vi "ClimbSequencer.vi"(7 "Reinit":bool) -> (0 "Climber Climbing":bool, 1 "Climber Power":dbl, 2 "Climber Pin":bool, 3 "PTO":bool, 4 "Climber Step":string)   [LabVIEW 2019]
uses:
  dsinstructions.vi
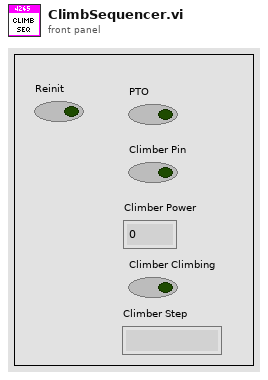
[diagram p1: front panel]
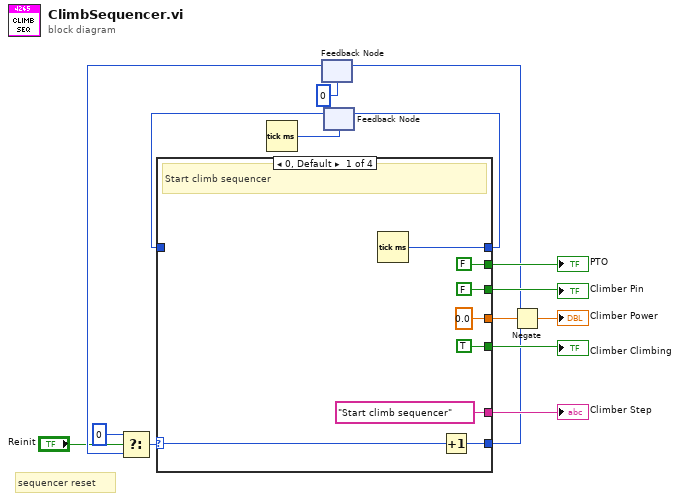
[diagram p0: block diagram]
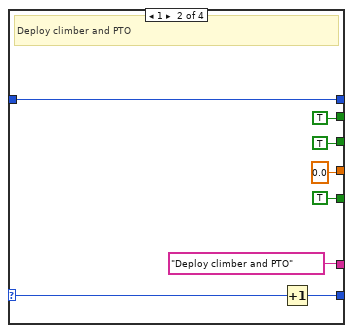
[diagram p2: hidden frame]
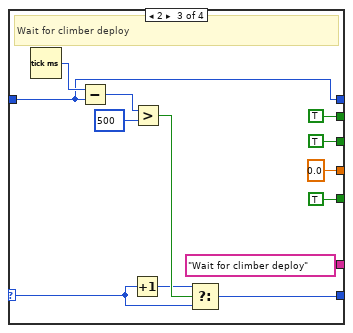
[diagram p3: hidden frame]
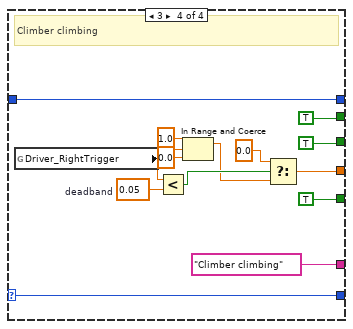
[diagram p4: hidden frame]
diagram:
  # "sequencer reset"
  n1 = Tick Count (ms)() -> (millisecond timer value=w6:u32)
  n2 = feedback #1(0) -> (w12:i32)
  n3 = Select(t=0, s="Reinit", f=w12) -> (s? t:f=w14:i32)
  n4 = feedback #2(w6) -> (w5:u32)
  n5 = case shown="0, Default" w14 {
    selector: w14 -> [w21 w31 w40 w57]
    tunnel: [w20 w26 w38 w57] -> w1
    tunnel: ["Start climb sequencer" "Deploy climber and PTO" "Wait for climber deploy" "Climber climbing"] -> w3
    tunnel: [w23 w27 w37 w56] -> w4
    tunnel: w5 -> [_ w27 w37 w56]
    tunnel: [0.0 ("Climber_Power") 0.0 ("Climber_Power") 0.0 ("Climber_Power") w52] -> w7
    tunnel: [FALSE TRUE TRUE TRUE] -> w8
    tunnel: [FALSE TRUE TRUE TRUE] -> w9
    tunnel: [TRUE TRUE TRUE TRUE] -> w10
    frame 0, Default {
      # "Start climb sequencer"
      n6 = Tick Count (ms)() -> (millisecond timer value=w23:u32)
      n7 = Increment(x=w21) -> (x+1=w20:i32)
    }
    frame 1 {
      # "Deploy climber and PTO"
      n8 = Increment(x=w31) -> (x+1=w26:i32)
    }
    frame 2 {
      # "Wait for climber deploy"
      n9 = Tick Count (ms)() -> (millisecond timer value=w44:u32)
      n10 = Subtract(x=w44, y=w37) -> (x-y=w43:u32)
      n11 = Increment(x=w40) -> (x+1=w39:i32)
      n12 = Greater?(x=w43, y=u32 500) -> (0:w41:bool)
      n13 = Select(t=w39, s=w41, f=w40) -> (s? t:f=w38:i32)
    }
    frame 3 {
      w49 = 0.05  # deadband
      # "Climber climbing"
      n14 = global read "dsinstructions.vi" "Driver_RightTrigger"() -> (w47:dbl)
      n15 = Less?(x=w47, y=w49) -> (x < y?=w51:bool)
      n16 = In Range and Coerce(upper limit=1.0, x=w47, lower limit=0.0) -> (coerced(x)=w48:dbl)  [unwired: 1 out]
      n17 = Select(t=0.0, s=w51, f=w48) -> (s? t:f=w52:dbl)
    }
  }
  "Climber Climbing" <- w10
  "Climber Pin" <- w9
  "PTO" <- w8
  "Climber Step" <- w3
  n18 = feedback-in #1(w1) -> ()
  n19 = feedback-in #2(w4) -> ()
  n20 = Negate(x=w7) -> (-x=→"Climber Power":dbl)
